vi "Begin.vi"(8 "error in":errorcluster) -> (0 "error out":errorcluster)   [LabVIEW 2018]
doc: "Called before other user functions, this VI is expected to open initial I/O refnums, load in file data, and do all program initialization. Notice that the <B>error out</B> terminal is simply used for data flow. Wiring it to other structures or subVIs ensures that this VI runs first."
uses:
  <vilib>/Rock Robotics/WPI/DriverStation/WPI_DriverStationRobotMode2.ctl
  <vilib>/Rock Robotics/SystemInterfaces/DIO/FPGA_DIOChannel.ctl
  <vilib>/Rock Robotics/WPI/Joystick/WPI_JoystickDeviceEnum.ctl
  <vilib>/Rock Robotics/WPI/Solenoid/WPI_SolenoidChannel.ctl
  <vilib>/Rock Robotics/WPI/ThirdParty/Phoenix-LabVIEW/Motor Controller/Controls/CTRE_Phoenix_MotorControl_FeedbackDevice.ctl
  Subsystems/Climb/climbStilt/climbStiltStateEnum.ctl
  Subsystems/Climb/climbStateEnum.ctl
  Subsystems/Climb/driveClimbStateEnum.ctl
  <vilib>/Rock Robotics/SystemInterfaces/i2clib/i2c_bus.ctl
  <vilib>/Rock Robotics/SystemInterfaces/AI/FPGA_AIChannel.ctl
  Subsystems/Drive/driveCommandEnum.ctl
  Subsystems/HatchPanel/hatchPanelNotifierCluster.ctl
  Subsystems/HatchPanel/hatchPanelEnum.ctl
  Subsystems/Sensors/Limelight/LimelightModeEnum.ctl
  Subsystems/Cargo/cargoNotifier.ctl
  Subsystems/Cargo/cargoEnum.ctl
  Subsystems/LineAlignment/LineAlignNotifier.ctl
  Subsystems/Drive/gear notifier.ctl
  Robot Global Data.vi
  <vilib>/Rock Robotics/WPI/Solenoid/WPI_SolenoidOpenSingle.vi
  <vilib>/Rock Robotics/WPI/ThirdParty/Phoenix-LabVIEW/Pigeon IMU/CTRE_PigeonIMU_Open_TalonSRX.vi
  <vilib>/Rock Robotics/WPI/Utilities/WPI_GetSetVariantRefNum.vi
panel:
  in  "Continuous Current Limit (Amps)":i32=32
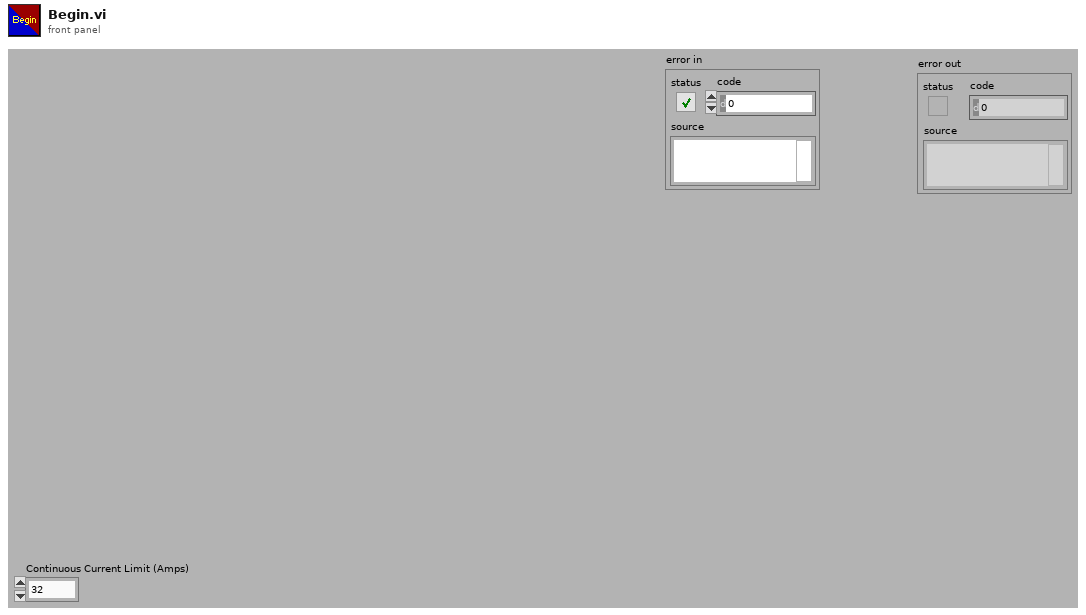
[diagram p1: front panel]
types:
  T1 = typedef "FPGA_DIOChannel.ctl" = enum8{"DIO 0", "DIO 1", "DIO 2", "DIO 3", "DIO 4", "DIO 5", "DIO 6", "DIO 7", "DIO 8", "DIO 9", "DIO MXP 0", "DIO MXP 1", "DIO MXP 2", "DIO MXP 3", "DIO MXP 4", "DIO MXP 5", "DIO MXP 6", "DIO MXP 7", "DIO MXP 8", "DIO MXP 9", "DIO MXP 10", "DIO MXP 11", "DIO MXP 12", "DIO MXP 13", "DIO MXP 14", "DIO MXP 15", "SPI Port CS1", "SPI Port CS2", "SPI Port CS3", "SPI Port MISO", "SPI Port MOSI", "Invalid"}
  T2 = typedef "gear notifier.ctl" = cluster{"High Gear?":bool, "Low Gear?":bool}
  T3 = typedef "LineAlignNotifier.ctl" = cluster{"skip 1":bool, "skip 2":bool, "LineAlign?":bool}
  T4 = typedef "cargoNotifier.ctl" = cluster{"Cargo State":T5, "Rocket?":bool, "Shoot":bool}
  T5 = typedef "cargoEnum.ctl" = enum16{"do nothing", "rocket right", "rocket left", "cargo ship left", "cargo ship right"}
  T6 = typedef "LimelightModeEnum.ctl" = enum16{"SA - Front", "SA - Rear", "SA - Side by Side", "Vision Processing"}
  T7 = typedef "WPI_JoystickDeviceEnum.ctl" = enum16{"USB 0", "USB 1", "USB 2", "USB 3", "USB 4", "USB 5"}
  T8 = typedef "WPI_SolenoidChannel.ctl" = enum8{"Solenoid 0", "Solenoid 1", "Solenoid 2", "Solenoid 3", "Solenoid 4", "Solenoid 5", "Solenoid 6", "Solenoid 7", "Invalid"}
  T9 = typedef "hatchPanelNotifierCluster.ctl" = cluster{"Hatch Panel State":T10, "Mechanism Motion":bool, "Gathering Claw Motion":bool, "Scoring Claw Motion":bool}
  T10 = typedef "hatchPanelEnum.ctl" = enum16{"do nothing", "State Machine", "Retracted Closed", "Retracted Open", "Extended Closed", "Extended Open"}
  T11 = typedef "driveCommandEnum.ctl" = enum16{"doNothing", "Manuel", "Teleop", "Follow Path", "Move to Target", "Climb", "Line Align", "Rotate180", "LoadingStation->CargoShip", "Sonar Brake", "LLCushion"}
  T12 = typedef "FPGA_AIChannel.ctl" = enum8{"AI 0", "AI 1", "AI 2", "AI 3", "AI MXP 0", "AI MXP 1", "AI MXP 2", "AI MXP 3", "Invalid"}
  T13 = typedef "i2c_bus.ctl" = enum16{"I2C On-Board", "I2C MXP", "Invalid"}
  T14 = enum32{"P0", "P1", "P2", "P3", "P4", "P5", "P6", "P7"}
  T15 = enum8{"ConfigMode", "AccOnly", "MagOnly", "GyroOnly", "AccMag", "AccGyro", "MagGyro", "AMG", "IMU", "Compass", "M4G", "NDOF_FMC_OFF", "NDOF"}
  T16 = typedef "driveClimbStateEnum.ctl" = enum16{"Do Nothing", "Drive Forward"}
  T17 = typedef "climbStateEnum.ctl" = enum16{"doNothing", "Auto Mode", "Safely Lower"}
  T18 = typedef "climbStiltStateEnum.ctl" = enum16{"doNothing", "Start/Safely Lower Both", "Both Extend", "Front Retract", "Both Retract"}
  T19 = typedef "CTRE_Phoenix_MotorControl_FeedbackDevice.ctl" = i8
  T20 = typedef "WPI_DriverStationRobotMode2.ctl" = enum16{"Autonomous Disabled", "Autonomous Enabled", "Teleop Disabled", "Teleop Enabled", "Disconnected", "Finish", "Test Disabled", "Test Enabled", "Emergency Stopped"}
  T21 = typedef "WPI_MotorControlDeviceRef.ctl" = cluster{"DeviceStatus":errorcluster, "Type":T22, "PWM":cluster{"PWM Channel":T23, "DeadBand":T24}, "CAN":cluster{"Device Number":u8, "SetOutput VI Ref":variant, "GetOutput VI Ref":variant, "Enable VI Ref":variant, "Disable VI Ref":variant, "Data":variant}, "Invert":bool, "DIO PWM":cluster{"PWM \"Enable\" Channel":T23, "DIOChannel":T1, "PWM Rate":dbl}}
  T22 = typedef "WPI_MotorControlType.ctl" = enum16{"PWM", "CAN", "DIO PWM"}
  T23 = typedef "FPGA_DIOPWMChannel.ctl" = enum8{"PWM 0", "PWM 1", "PWM 2", "PWM 3", "PWM 4", "PWM 5", "PWM 6", "PWM 7", "PWM 8", "PWM 9", "PWM MXP 0", "PWM MXP 1", "PWM MXP 2", "PWM MXP 3", "PWM MXP 4", "PWM MXP 5", "PWM MXP 6", "PWM MXP 7", "PWM MXP 8", "PWM MXP 9", "Invalid"}
  T24 = typedef "WPI_PWMDeadband.ctl" = cluster{"Name":string, "maxPositivePwm":i32, "minPositivePwm":i32, "centerPwm":i32, "maxNegativePwm":i32, "minNegativePwm":i32, "angularRange":u16}
  T25 = typedef "WPI_JoystickDevRef.ctl" = cluster{"Device":T7}
  T26 = typedef "CTRE_PigeonIMU_DeviceRef.ctl" = cluster{"DeviceStatus":errorcluster, "Device Number":u8, "Type":T27, "Device ID":u32, "Handle":u64, "UsageFrame":u32, "Library Path":path}
  T27 = typedef "CTRE_PigeonIMU_ConnectionType.ctl" = u32
  T28 = typedef "WPI_SolenoidDevRef.ctl" = cluster{"DevStatus":errorcluster, "Pneumatics Control Module":u8, "Forward Solenoid Channel":T8, "Reverse Solenoid Channel":T8}
  T29 = typedef "WPI_CompressorDevRef.ctl" = cluster{"DevStatus":errorcluster, "Pneumatics Control Module":u8}
  T30 = typedef "WPI_DigitalInputDevRef.ctl" = cluster{"DevStatus":errorcluster, "DIO Channel":T1}
  T31 = typedef "WPI_AnalogChannelDevRef.ctl" = cluster{"DevStatus":errorcluster, "Analog Channel":T12}
  T32 = typedef "ImuDevRef.ctl" = cluster{"I2CDevRef":T33, "Valid Cal File?":bool}
  T33 = typedef "WPI_I2CDevRef.ctl" = cluster{"DevStatus":errorcluster, "Device Address":u8, "Handle":i32, "I2C Bus":T13}
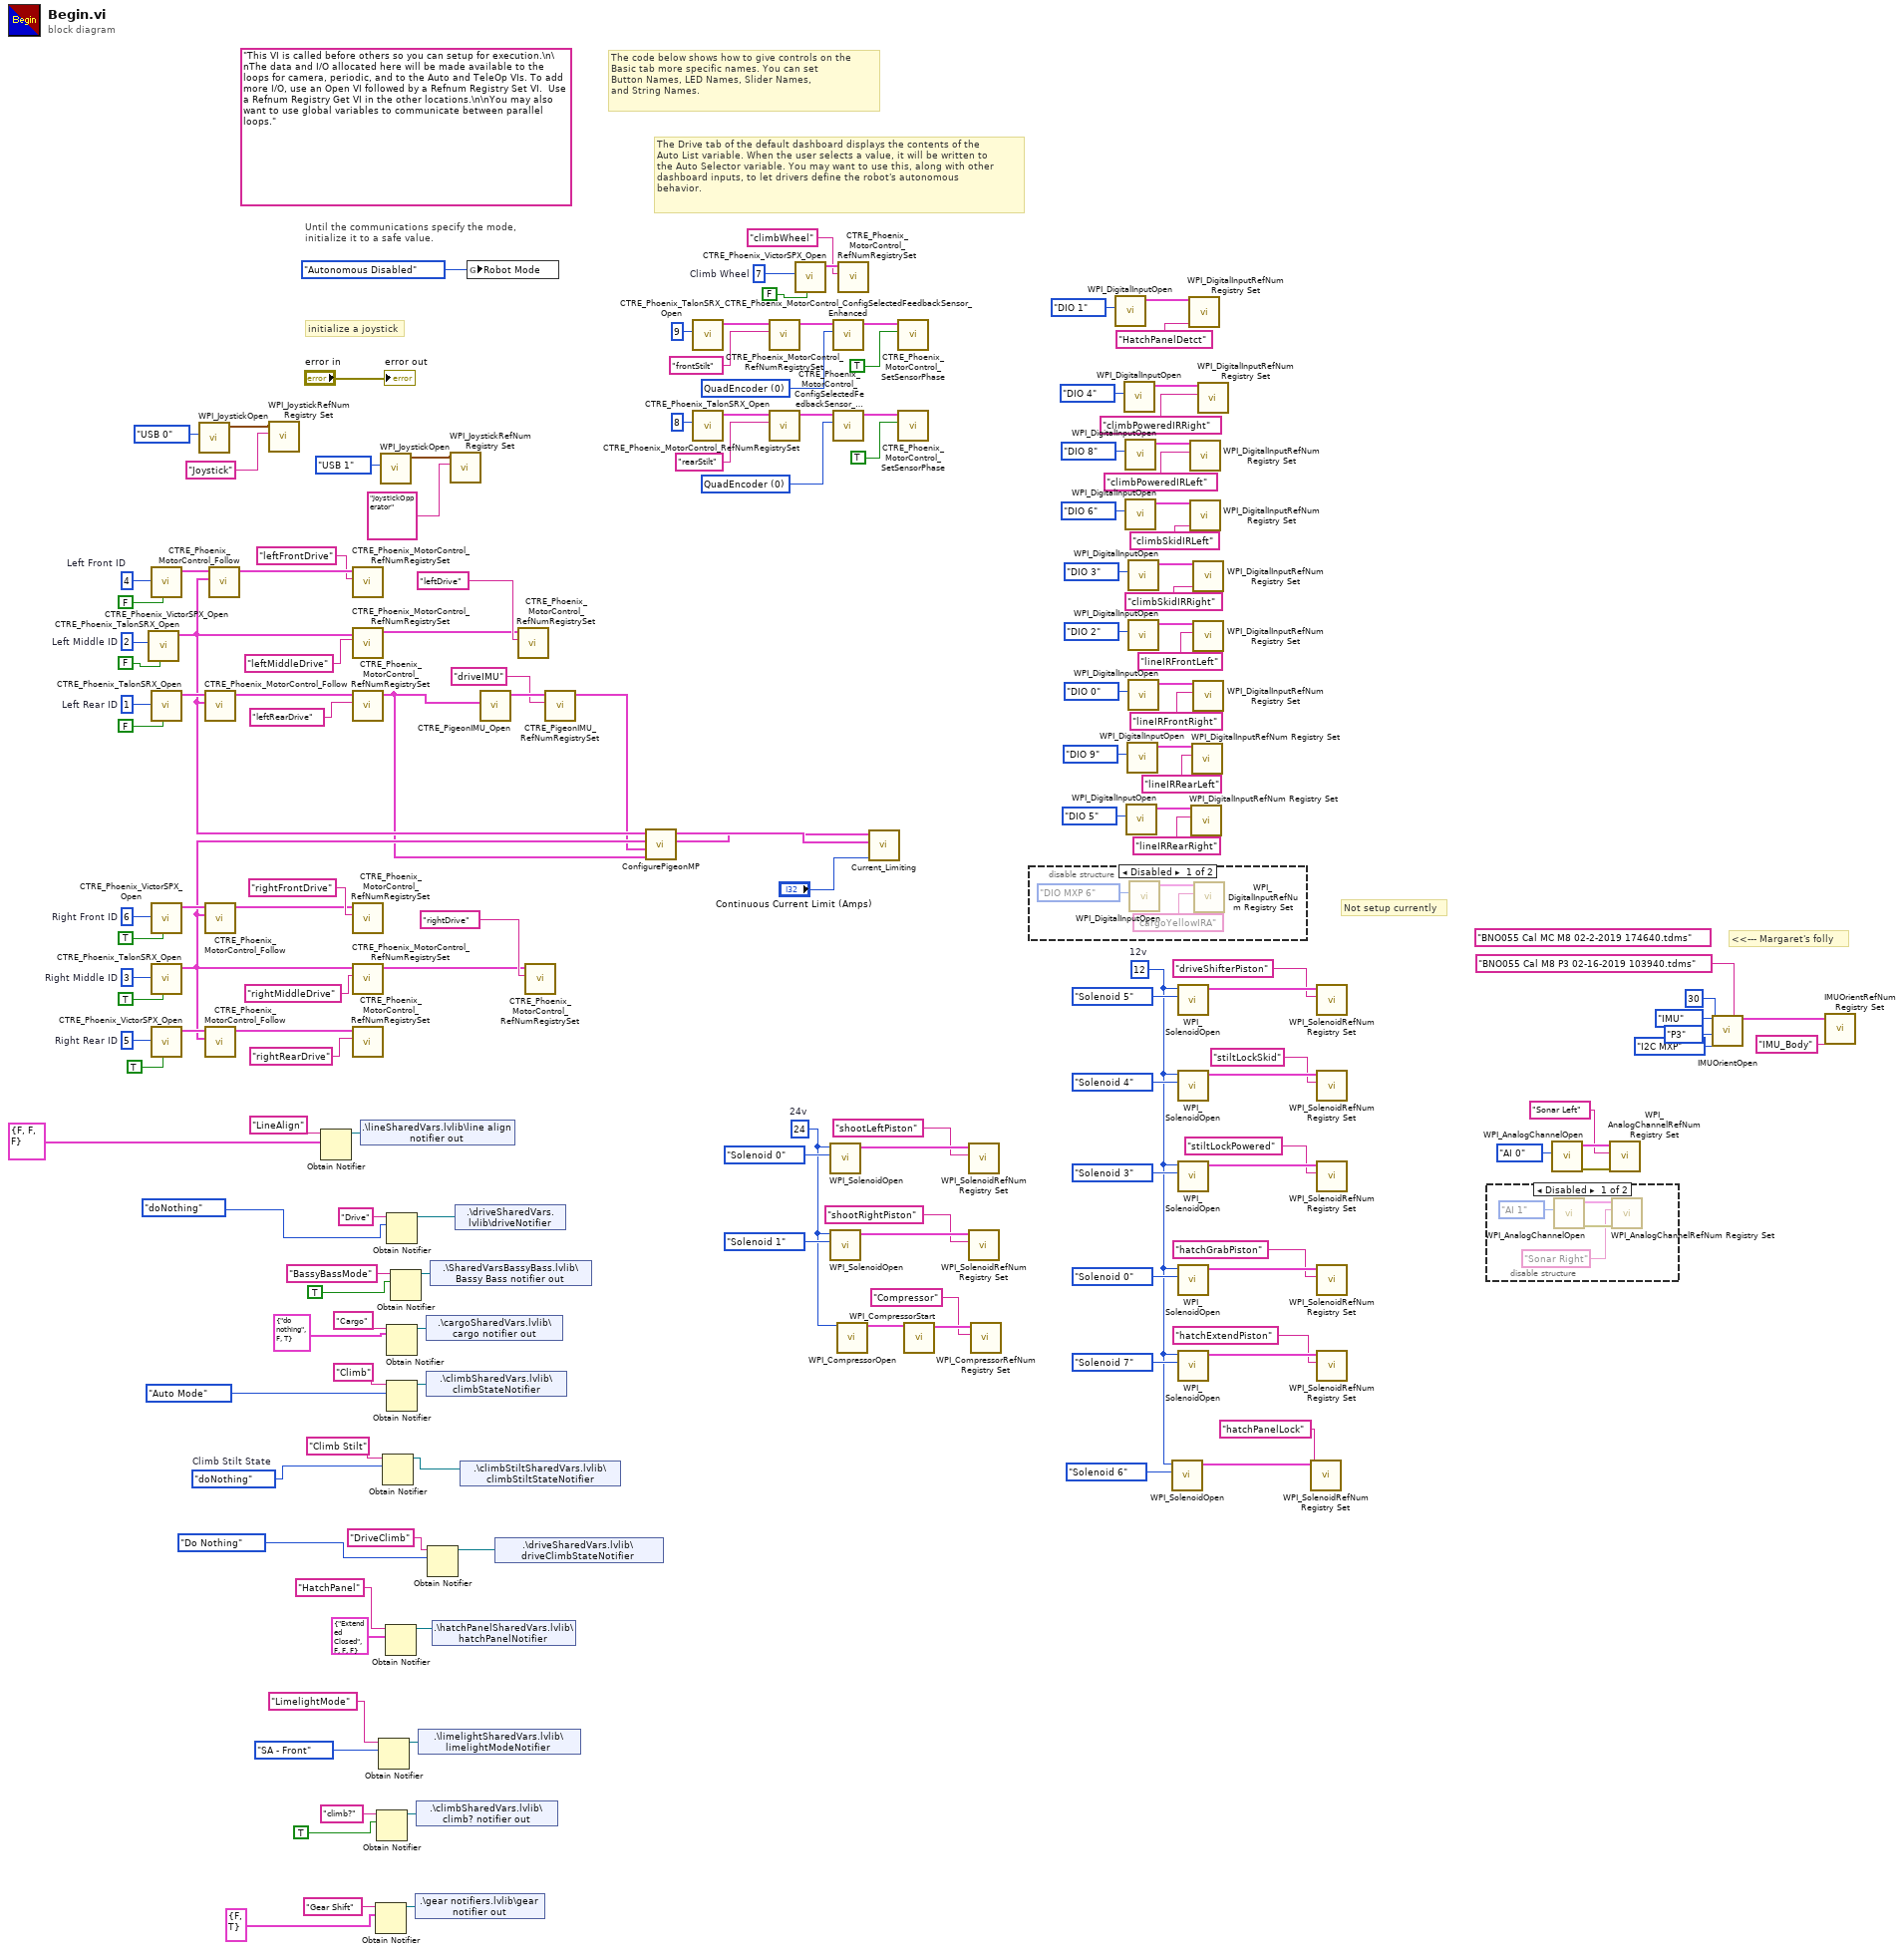
[diagram p0: block diagram]
diagram:
  w66 = u8 1  # Left Rear ID
  w56 = u8 2  # Left Middle ID
  w68 = u8 4  # Left Front ID
  w69 = u8 5  # Right Rear ID
  w71 = u8 3  # Right Middle ID
  w73 = u8 6  # Right Front ID
  (unwired) "BNO055 Cal MC M8 02-2-2019 174640.tdms" ("Stored Cal File")
  w91 = climbStiltStateEnum."doNothing"  # Climb Stilt State
  w97 = T19 0 items=["QuadEncoder"=0, "Analog"=2, "Tachometer"=4, "Pulse Width Encoded Position"=8, "Sensor Sum (S0 + S1)"=9, "Sensor Difference (D0 - D1)"=10, "Remote Source 0"=11, "Remote Source 1"=12, "Software Emulated"=15] ("Feedback Device")
  w98 = T19 0 items=["QuadEncoder"=0, "Analog"=2, "Tachometer"=4, "Pulse Width Encoded Position"=8, "Sensor Sum (S0 + S1)"=9, "Sensor Difference (D0 - D1)"=10, "Remote Source 0"=11, "Remote Source 1"=12, "Software Emulated"=15] ("Feedback Device")
  w110 = u8 7  # Climb Wheel
  w30 = u8 12  # 12v
  w26 = u8 24  # 24v
  (unwired) "This VI is called before others so you can setup for execution.\n\nThe data and I/O allocated here will be made available to the loops for camera, periodic, and to the Auto and TeleOp VIs. To add more I/O, use an Open VI followed by a Refnum Registry Set VI.  Use a Refnum Registry Get VI in the other locations.\n\nYou may also want to use global variables to communicate between parallel loops."
  # "<<--- Margaret's folly"
  # "Not setup currently"
  # "The Drive tab of the default dashboard displays the contents of the\nAuto List variable. When the user selects a value, it will be written to\nthe Auto Selector variable. You may want to use this, along with other\ndashboard inputs, to let drivers define the robot's autonomous\nbehavior."
  # "The code below shows how to give controls on the\nBasic tab more specific names. You can set\nButton Names, LED Names, Slider Names,\nand String Names."
  # "initialize a joystick"
  # "Until the communications specify the mode,\ninitialize it to a safe value."
  n1 = call <vilib>:"CTRE_Phoenix_TalonSRX_Open.vi"("Invert"=FALSE, "Device Number"=w56) -> ("CAN Talon SRX Ref"=w46:T21)  [unwired: 8 in, 1 out]
  n2 = call <vilib>:"CTRE_Phoenix_VictorSPX_Open.vi"("Invert"=FALSE, "Device Number"=w68) -> ("CAN Talon SRX Ref"=w51:T21)  [unwired: 8 in, 1 out]
  n3 = call <vilib>:"CTRE_Phoenix_TalonSRX_Open.vi"("Invert"=FALSE, "Device Number"=w66) -> ("CAN Talon SRX Ref"=w63:T21)  [unwired: 8 in, 1 out]
  n4 = call <vilib>:"CTRE_Phoenix_VictorSPX_Open.vi"("Invert"=TRUE, "Device Number"=w73) -> ("CAN Talon SRX Ref"=w50:T21)  [unwired: 8 in, 1 out]
  n5 = call <vilib>:"CTRE_Phoenix_TalonSRX_Open.vi"("Invert"=TRUE, "Device Number"=w71) -> ("CAN Talon SRX Ref"=w43:T21)  [unwired: 8 in, 1 out]
  n6 = call <vilib>:"CTRE_Phoenix_VictorSPX_Open.vi"("Invert"=TRUE, "Device Number"=w69) -> ("CAN Talon SRX Ref"=w64:T21)  [unwired: 8 in, 1 out]
  n7 = call <vilib>:"WPI_JoystickOpen.vi"("JoystickDevice"=WPI_JoystickDeviceEnum."USB 0") -> ("JoystickDevRef"=w134:T25)  [unwired: 10 in]
  n8 = call <vilib>:"CTRE_Phoenix_MotorControl_Follow.vi"("Master Controller to Follow"=w46, "PhoenixMotorControlDevRef"=w63) -> ("PhoenixMotorControlDevRef"=w62:T21)  [unwired: 8 in, 1 out]
  n9 = call <vilib>:"CTRE_Phoenix_MotorControl_Follow.vi"("Master Controller to Follow"=w43, "PhoenixMotorControlDevRef"=w50) -> ("PhoenixMotorControlDevRef"=w49:T21)  [unwired: 8 in, 1 out]
  n10 = call <vilib>:"CTRE_Phoenix_MotorControl_Follow.vi"("Master Controller to Follow"=w43, "PhoenixMotorControlDevRef"=w64) -> ("PhoenixMotorControlDevRef"=w61:T21)  [unwired: 8 in, 1 out]
  n11 = call <vilib>:"CTRE_Phoenix_MotorControl_Follow.vi"("Master Controller to Follow"=w46, "PhoenixMotorControlDevRef"=w51) -> ("PhoenixMotorControlDevRef"=w52:T21)  [unwired: 8 in, 1 out]
  n12 = call <vilib>:"WPI_JoystickRefNum Registry Set.vi"("refnum name"="Joystick", "JoystickDevRef"=w134) -> ()  [unwired: 8 in, 2 out]
  n13 = Obtain Notifier(name (unnamed)="LineAlign", notification data type=T3 {"skip 1"=FALSE, "skip 2"=FALSE, "LineAlign?"=FALSE}) -> (notifier out=w13:refnum<notifier>)  [unwired: 2 in, 2 out]
  n14 = call <vilib>:"CTRE_Phoenix_MotorControl_RefNumRegistrySet.vi"("refnum name"="leftFrontDrive", "PhoenixMotorControlDevRef"=w52) -> ()  [unwired: 8 in, 2 out]
  n15 = call <vilib>:"CTRE_Phoenix_MotorControl_RefNumRegistrySet.vi"("refnum name"="leftMiddleDrive", "PhoenixMotorControlDevRef"=w46) -> ("PhoenixMotorControlDevRef"=w40:T21)  [unwired: 8 in, 1 out]
  n16 = call <vilib>:"CTRE_Phoenix_MotorControl_RefNumRegistrySet.vi"("refnum name"="leftRearDrive", "PhoenixMotorControlDevRef"=w62) -> ("PhoenixMotorControlDevRef"=w41:T21)  [unwired: 8 in, 1 out]
  n17 = call <vilib>:"CTRE_Phoenix_MotorControl_RefNumRegistrySet.vi"("refnum name"="rightFrontDrive", "PhoenixMotorControlDevRef"=w49) -> ()  [unwired: 8 in, 2 out]
  n18 = call <vilib>:"CTRE_Phoenix_MotorControl_RefNumRegistrySet.vi"("refnum name"="rightMiddleDrive", "PhoenixMotorControlDevRef"=w43) -> ("PhoenixMotorControlDevRef"=w39:T21)  [unwired: 8 in, 1 out]
  n19 = call <vilib>:"CTRE_Phoenix_MotorControl_RefNumRegistrySet.vi"("refnum name"="rightRearDrive", "PhoenixMotorControlDevRef"=w61) -> ()  [unwired: 8 in, 2 out]
  n20 = shared-variable ".\\lineSharedVars.lvlib\\line align notifier out"(w13) -> ()  [unwired: 1 in, 1 out]
  n21 = Obtain Notifier(name (unnamed)="Gear Shift", notification data type=T2 {"High Gear?"=FALSE, "Low Gear?"=TRUE} ("Cluster")) -> (notifier out=w4:refnum<notifier>)  [unwired: 2 in, 2 out]
  n22 = Obtain Notifier(name (unnamed)="climb?", notification data type=TRUE ("create if not found? (T)")) -> (notifier out=w7:refnum<notifier>)  [unwired: 2 in, 2 out]
  n23 = Obtain Notifier(name (unnamed)="LimelightMode", notification data type=LimelightModeEnum."SA - Front" ("Enum")) -> (notifier out=w18:refnum<notifier>)  [unwired: 2 in, 2 out]
  n24 = call <vilib>:"WPI_JoystickOpen.vi"("JoystickDevice"=WPI_JoystickDeviceEnum."USB 1") -> ("JoystickDevRef"=w23:T25)  [unwired: 10 in]
  n25 = Obtain Notifier(name (unnamed)="Climb Stilt", notification data type=w91) -> (notifier out=w90:refnum<notifier>)  [unwired: 2 in, 2 out]
  n26 = Obtain Notifier(name (unnamed)="HatchPanel", notification data type=T9 {"Hatch Panel State"=enum."Extended Closed", "Mechanism Motion"=FALSE, "Gathering Claw Motion"=FALSE, "Scoring Claw Motion"=FALSE}) -> (notifier out=w33:refnum<notifier>)  [unwired: 2 in, 2 out]
  n27 = Obtain Notifier(name (unnamed)="Drive", notification data type=driveCommandEnum."doNothing" ("Drive Command Enum")) -> (notifier out=w159:refnum<notifier>)  [unwired: 2 in, 2 out]
  n28 = Obtain Notifier(name (unnamed)="Cargo", notification data type=T4 {"Cargo State"=enum."do nothing", "Rocket?"=FALSE, "Shoot"=TRUE}) -> (notifier out=w16:refnum<notifier>)  [unwired: 2 in, 2 out]
  n29 = Obtain Notifier(name (unnamed)="Climb", notification data type=climbStateEnum."Auto Mode" ("Climb State")) -> (notifier out=w88:refnum<notifier>)  [unwired: 2 in, 2 out]
  n30 = Obtain Notifier(name (unnamed)="BassyBassMode", notification data type=TRUE ("create if not found? (T)")) -> (notifier out=w10:refnum<notifier>)  [unwired: 2 in, 2 out]
  n31 = shared-variable ".\\gear notifiers.lvlib\\gear notifier out"(w4) -> ()  [unwired: 1 in, 1 out]
  n32 = shared-variable ".\\climbSharedVars.lvlib\\climb? notifier out"(w7) -> ()  [unwired: 1 in, 1 out]
  n33 = shared-variable ".\\limelightSharedVars.lvlib\\limelightModeNotifier"(w18) -> ()  [unwired: 1 in, 1 out]
  n34 = shared-variable ".\\cargoSharedVars.lvlib\\cargo notifier out"(w16) -> ()  [unwired: 1 in, 1 out]
  n35 = shared-variable ".\\climbSharedVars.lvlib\\climbStateNotifier"(w88) -> ()  [unwired: 1 in, 1 out]
  n36 = Obtain Notifier(name (unnamed)="DriveClimb", notification data type=driveClimbStateEnum."Do Nothing" ("Drive Climb State")) -> (notifier out=w85:refnum<notifier>)  [unwired: 2 in, 2 out]
  n37 = shared-variable ".\\SharedVarsBassyBass.lvlib\\Bassy Bass notifier out"(w10) -> ()  [unwired: 1 in, 1 out]
  n38 = shared-variable ".\\hatchPanelSharedVars.lvlib\\hatchPanelNotifier"(w33) -> ()  [unwired: 1 in, 1 out]
  n39 = call <vilib>:"WPI_JoystickRefNum Registry Set.vi"("refnum name"="JoystickOpperator", "JoystickDevRef"=w23) -> ()  [unwired: 8 in, 2 out]
  n40 = shared-variable ".\\driveSharedVars.lvlib\\driveNotifier"(w159) -> ()  [unwired: 1 in, 1 out]
  n41 = shared-variable ".\\climbStiltSharedVars.lvlib\\climbStiltStateNotifier"(w90) -> ()  [unwired: 1 in, 1 out]
  n42 = global write "Robot Global Data.vi" "Robot Mode"(WPI_DriverStationRobotMode2."Autonomous Disabled" ("Robot Mode")) -> ()
  n43 = call-poly <vilib>:"CTRE_PigeonIMU_Open.vi"("CAN Talon SRX Ref"=w41) -> ("PigeonIMUDevRef"=w48:T26)  [unwired: 9 in, 1 out]
  n44 = shared-variable ".\\driveSharedVars.lvlib\\driveClimbStateNotifier"(w85) -> ()  [unwired: 1 in, 1 out]
  n45 = call <vilib>:"CTRE_Phoenix_MotorControl_RefNumRegistrySet.vi"("refnum name"="leftDrive", "PhoenixMotorControlDevRef"=w40) -> ()  [unwired: 8 in, 2 out]
  n46 = call <vilib>:"CTRE_Phoenix_MotorControl_RefNumRegistrySet.vi"("refnum name"="rightDrive", "PhoenixMotorControlDevRef"=w39) -> ()  [unwired: 8 in, 2 out]
  n47 = call <vilib>:"CTRE_PigeonIMU_RefNumRegistrySet.vi"("refnum name"="driveIMU", "PigeonIMUDevRef"=w48) -> ("PigeonIMUDevRef"=w42:T26)  [unwired: 8 in, 1 out]
  n48 = call "ConfigurePigeonMP.vi"("Pigeon Talon"=w41, "Pigeon"=w42, "Right Side"=w43, "Left Side"=w46) -> ("Right Side"=w44:T21, "Left Side"=w45:T21)  [unwired: 5 in, 1 out]
  n49 = call <vilib>:"CTRE_Phoenix_TalonSRX_Open.vi"("Device Number"=u8 9) -> ("CAN Talon SRX Ref"=w104:T21)  [unwired: 9 in, 1 out]
  n50 = call <vilib>:"CTRE_Phoenix_TalonSRX_Open.vi"("Device Number"=u8 8) -> ("CAN Talon SRX Ref"=w103:T21)  [unwired: 9 in, 1 out]
  n51 = call <vilib>:"CTRE_Phoenix_MotorControl_RefNumRegistrySet.vi"("refnum name"="frontStilt", "PhoenixMotorControlDevRef"=w104) -> ("PhoenixMotorControlDevRef"=w100:T21)  [unwired: 8 in, 1 out]
  n52 = call <vilib>:"CTRE_Phoenix_MotorControl_RefNumRegistrySet.vi"("refnum name"="rearStilt", "PhoenixMotorControlDevRef"=w103) -> ("PhoenixMotorControlDevRef"=w99:T21)  [unwired: 8 in, 1 out]
  n53 = call <vilib>:"CTRE_Phoenix_VictorSPX_Open.vi"("Invert"=FALSE, "Device Number"=w110) -> ("CAN Talon SRX Ref"=w108:T21)  [unwired: 8 in, 1 out]
  n54 = call-poly <vilib>:"WPI_SolenoidOpen.vi"("Solenoid Channel"=WPI_SolenoidChannel."Solenoid 0", "Pneumatics Control Module (0)"=w26) -> ("SolenoidDevRef"=w130:T28)  [unwired: 8 in, 1 out]
  n55 = call-poly <vilib>:"WPI_SolenoidOpen.vi"("Solenoid Channel"=WPI_SolenoidChannel."Solenoid 1", "Pneumatics Control Module (0)"=w26) -> ("SolenoidDevRef"=w127:T28)  [unwired: 8 in, 1 out]
  n56 = call <vilib>:"CTRE_Phoenix_MotorControl_ConfigSelectedFeedbackSensor_Enhanced.vi"("Feedback Device"=w98, "PhoenixMotorControlDevRef"=w100) -> ("PhoenixMotorControlDevRef"=w95:T21)  [unwired: 8 in, 1 out]
  n57 = call <vilib>:"CTRE_Phoenix_MotorControl_ConfigSelectedFeedbackSensor_Enhanced.vi"("Feedback Device"=w97, "PhoenixMotorControlDevRef"=w99) -> ("PhoenixMotorControlDevRef"=w96:T21)  [unwired: 8 in, 1 out]
  n58 = call <vilib>:"WPI_CompressorOpen.vi"("Pneumatics Control Module (0)"=w26) -> ("CompressorDevRef"=w28:T29)  [unwired: 13 in, 1 out]
  n59 = call <vilib>:"CTRE_Phoenix_MotorControl_RefNumRegistrySet.vi"("refnum name"="climbWheel", "PhoenixMotorControlDevRef"=w108) -> ()  [unwired: 8 in, 2 out]
  n60 = call "Current_Limiting.vi"("Continuous Current Limit (Amps)"="Continuous Current Limit (Amps)", "Left PhoenixMotorControlDevRef"=w45, "Right PhoenixMotorControlDevRef"=w44) -> ()  [unwired: 9 in]
  n61 = call <vilib>:"CTRE_Phoenix_MotorControl_SetSensorPhase.vi"("PhaseSensor"=TRUE, "PhoenixMotorControlDevRef"=w95) -> ()  [unwired: 8 in, 2 out]
  n62 = call <vilib>:"CTRE_Phoenix_MotorControl_SetSensorPhase.vi"("PhaseSensor"=TRUE, "PhoenixMotorControlDevRef"=w96) -> ()  [unwired: 8 in, 2 out]
  n63 = call <vilib>:"WPI_CompressorStart.vi"("CompressorDevRef"=w28) -> ("CompressorDevRef"=w27:T29)  [unwired: 9 in, 1 out]
  n64 = call <vilib>:"WPI_SolenoidRefNum Registry Set.vi"("refnum name"="shootLeftPiston", "SolenoidDevRef"=w130) -> ()  [unwired: 8 in, 2 out]
  n65 = call <vilib>:"WPI_SolenoidRefNum Registry Set.vi"("refnum name"="shootRightPiston", "SolenoidDevRef"=w127) -> ()  [unwired: 8 in, 2 out]
  n66 = call <vilib>:"WPI_CompressorRefNum Registry Set.vi"("refnum name"="Compressor", "CompressorDevRef"=w27) -> ()  [unwired: 8 in, 2 out]
  n67 = disable-structure shown="Disabled" {
    frame Disabled {
      n68 = call <vilib>:"WPI_DigitalInputOpen.vi"("DIO Channel"=FPGA_DIOChannel."DIO MXP 6") -> ("DigitalInputDevRef"=w168:T30)  [unwired: 9 in, 1 out]
      n69 = call <vilib>:"WPI_DigitalInputRefNum Registry Set.vi"("refnum name"="cargoYellowIRA", "DigitalInputDevRef"=w168) -> ()  [unwired: 8 in, 2 out]
    }
    frame Enabled {
    }
  }
  n70 = call <vilib>:"WPI_DigitalInputOpen.vi"("DIO Channel"=FPGA_DIOChannel."DIO 1") -> ("DigitalInputDevRef"=w3:T30)  [unwired: 9 in, 1 out]
  n71 = call <vilib>:"WPI_DigitalInputOpen.vi"("DIO Channel"=FPGA_DIOChannel."DIO 4") -> ("DigitalInputDevRef"=w158:T30)  [unwired: 9 in, 1 out]
  n72 = call <vilib>:"WPI_DigitalInputOpen.vi"("DIO Channel"=FPGA_DIOChannel."DIO 8") -> ("DigitalInputDevRef"=w156:T30)  [unwired: 9 in, 1 out]
  n73 = call <vilib>:"WPI_DigitalInputOpen.vi"("DIO Channel"=FPGA_DIOChannel."DIO 6") -> ("DigitalInputDevRef"=w152:T30)  [unwired: 9 in, 1 out]
  n74 = call <vilib>:"WPI_DigitalInputOpen.vi"("DIO Channel"=FPGA_DIOChannel."DIO 5") -> ("DigitalInputDevRef"=w137:T30)  [unwired: 9 in, 1 out]
  n75 = call <vilib>:"WPI_DigitalInputOpen.vi"("DIO Channel"=FPGA_DIOChannel."DIO 9") -> ("DigitalInputDevRef"=w140:T30)  [unwired: 9 in, 1 out]
  n76 = call <vilib>:"WPI_DigitalInputOpen.vi"("DIO Channel"=FPGA_DIOChannel."DIO 3") -> ("DigitalInputDevRef"=w149:T30)  [unwired: 9 in, 1 out]
  n77 = call <vilib>:"WPI_DigitalInputOpen.vi"("DIO Channel"=FPGA_DIOChannel."DIO 2") -> ("DigitalInputDevRef"=w146:T30)  [unwired: 9 in, 1 out]
  n78 = call <vilib>:"WPI_DigitalInputOpen.vi"("DIO Channel"=FPGA_DIOChannel."DIO 0") -> ("DigitalInputDevRef"=w143:T30)  [unwired: 9 in, 1 out]
  n79 = call-poly <vilib>:"WPI_SolenoidOpen.vi"("Solenoid Channel"=WPI_SolenoidChannel."Solenoid 6", "Pneumatics Control Module (0)"=w30) -> ("SolenoidDevRef"=w31:T28)  [unwired: 8 in, 1 out]
  n80 = call-poly <vilib>:"WPI_SolenoidOpen.vi"("Solenoid Channel"=WPI_SolenoidChannel."Solenoid 5", "Pneumatics Control Module (0)"=w30) -> ("SolenoidDevRef"=w124:T28)  [unwired: 8 in, 1 out]
  n81 = call-poly <vilib>:"WPI_SolenoidOpen.vi"("Solenoid Channel"=WPI_SolenoidChannel."Solenoid 4", "Pneumatics Control Module (0)"=w30) -> ("SolenoidDevRef"=w121:T28)  [unwired: 8 in, 1 out]
  n82 = call-poly <vilib>:"WPI_SolenoidOpen.vi"("Solenoid Channel"=WPI_SolenoidChannel."Solenoid 3", "Pneumatics Control Module (0)"=w30) -> ("SolenoidDevRef"=w118:T28)  [unwired: 8 in, 1 out]
  n83 = call-poly <vilib>:"WPI_SolenoidOpen.vi"("Solenoid Channel"=WPI_SolenoidChannel."Solenoid 0", "Pneumatics Control Module (0)"=w30) -> ("SolenoidDevRef"=w115:T28)  [unwired: 8 in, 1 out]
  n84 = call-poly <vilib>:"WPI_SolenoidOpen.vi"("Solenoid Channel"=WPI_SolenoidChannel."Solenoid 7", "Pneumatics Control Module (0)"=w30) -> ("SolenoidDevRef"=w112:T28)  [unwired: 8 in, 1 out]
  n85 = call <vilib>:"WPI_DigitalInputRefNum Registry Set.vi"("refnum name"="HatchPanelDetct", "DigitalInputDevRef"=w3) -> ()  [unwired: 8 in, 2 out]
  n86 = call <vilib>:"WPI_DigitalInputRefNum Registry Set.vi"("refnum name"="climbPoweredIRLeft", "DigitalInputDevRef"=w156) -> ()  [unwired: 8 in, 2 out]
  n87 = call <vilib>:"WPI_DigitalInputRefNum Registry Set.vi"("refnum name"="climbSkidIRLeft", "DigitalInputDevRef"=w152) -> ()  [unwired: 8 in, 2 out]
  n88 = call <vilib>:"WPI_DigitalInputRefNum Registry Set.vi"("refnum name"="lineIRRearRight", "DigitalInputDevRef"=w137) -> ()  [unwired: 8 in, 2 out]
  n89 = call <vilib>:"WPI_DigitalInputRefNum Registry Set.vi"("refnum name"="lineIRRearLeft", "DigitalInputDevRef"=w140) -> ()  [unwired: 8 in, 2 out]
  n90 = call <vilib>:"WPI_DigitalInputRefNum Registry Set.vi"("refnum name"="climbSkidIRRight", "DigitalInputDevRef"=w149) -> ()  [unwired: 8 in, 2 out]
  n91 = call <vilib>:"WPI_DigitalInputRefNum Registry Set.vi"("refnum name"="lineIRFrontLeft", "DigitalInputDevRef"=w146) -> ()  [unwired: 8 in, 2 out]
  n92 = call <vilib>:"WPI_DigitalInputRefNum Registry Set.vi"("refnum name"="lineIRFrontRight", "DigitalInputDevRef"=w143) -> ()  [unwired: 8 in, 2 out]
  n93 = call <vilib>:"WPI_DigitalInputRefNum Registry Set.vi"("refnum name"="climbPoweredIRRight", "DigitalInputDevRef"=w158) -> ()  [unwired: 8 in, 2 out]
  n94 = call <vilib>:"WPI_SolenoidRefNum Registry Set.vi"("refnum name"="hatchPanelLock", "SolenoidDevRef"=w31) -> ()  [unwired: 8 in, 2 out]
  n95 = call <vilib>:"WPI_SolenoidRefNum Registry Set.vi"("refnum name"="driveShifterPiston", "SolenoidDevRef"=w124) -> ()  [unwired: 8 in, 2 out]
  n96 = call <vilib>:"WPI_SolenoidRefNum Registry Set.vi"("refnum name"="stiltLockSkid", "SolenoidDevRef"=w121) -> ()  [unwired: 8 in, 2 out]
  n97 = call <vilib>:"WPI_SolenoidRefNum Registry Set.vi"("refnum name"="stiltLockPowered", "SolenoidDevRef"=w118) -> ()  [unwired: 8 in, 2 out]
  n98 = call <vilib>:"WPI_SolenoidRefNum Registry Set.vi"("refnum name"="hatchGrabPiston", "SolenoidDevRef"=w115) -> ()  [unwired: 8 in, 2 out]
  n99 = call <vilib>:"WPI_SolenoidRefNum Registry Set.vi"("refnum name"="hatchExtendPiston", "SolenoidDevRef"=w112) -> ()  [unwired: 8 in, 2 out]
  n100 = disable-structure shown="Disabled" {
    frame Disabled {
      n101 = call <vilib>:"WPI_AnalogChannelOpen.vi"("Analog Channel"=FPGA_AIChannel."AI 1") -> ("error out"=w172:errorcluster, "AIDeviceRef"=w171:T31)  [unwired: 9 in]
      n102 = call <vilib>:"WPI_AnalogChannelRefNum Registry Set.vi"("error in (no error)"=w172, "refnum name"="Sonar Right", "AIDeviceRef"=w171) -> ()  [unwired: 7 in, 2 out]
    }
    frame Enabled {
    }
  }
  n103 = call <vilib>:"WPI_AnalogChannelOpen.vi"("Analog Channel"=FPGA_AIChannel."AI 0") -> ("error out"=w77:errorcluster, "AIDeviceRef"=w76:T31)  [unwired: 9 in]
  n104 = call <vilib>:"WPI_AnalogChannelRefNum Registry Set.vi"("error in (no error)"=w77, "refnum name"="Sonar Left", "AIDeviceRef"=w76) -> ()  [unwired: 7 in, 2 out]
  n105 = call <userlib>:"IMUOrientOpen.vi"("Op Mode"=T15."IMU", "Stored Cal File"="BNO055 Cal M8 P3 02-16-2019 103940.tdms", "Placement"=T14."P3", "I2C Bus"=i2c_bus."I2C MXP", "Status delay"=30) -> ("IMU Dev Ref"=w84:T32)  [unwired: 4 in, 6 out]
  n106 = call <userlib>:"IMUOrientRefNum Registry Set.vi"("refnum name"="IMU_Body", "IMUDevRef in"=w84) -> ()  [unwired: 8 in, 2 out]
  "error out" <- "error in"
